vi "Set speed DSP402.vi"(8 "error in (no error)":errorcluster, 10 "RpM":i16, 11 "DSP402 in":refnum<class "DSP402.lvclass">) -> (0 "error out":errorcluster, 3 "DSP402 out":refnum<class "DSP402.lvclass">)   [LabVIEW 2026, in "canopen_.lvlib" / "DSP402.lvclass"]
uses:
  DSP402.lvclass
  DSP402.lvclass/DSP402.ctl
  CANopen/Multiplexor.ctl
  CANopen Master.lvlib
  Download DSP402 (U32).vi
  Download DSP402 (U16).vi
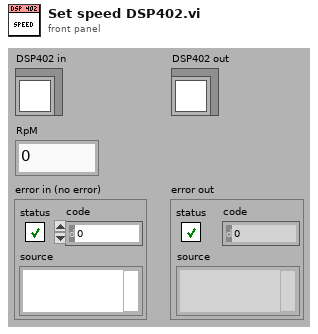
[diagram p1: front panel]
types:
  T1 = typedef "canopen.lvlib/DSP402.lvclass/DriveMode.ctl" = i8
  T2 = typedef "CANopen Master.lvlib/Multiplexor.ctl" = cluster{"Index":u16, "Sub-Index":i16}
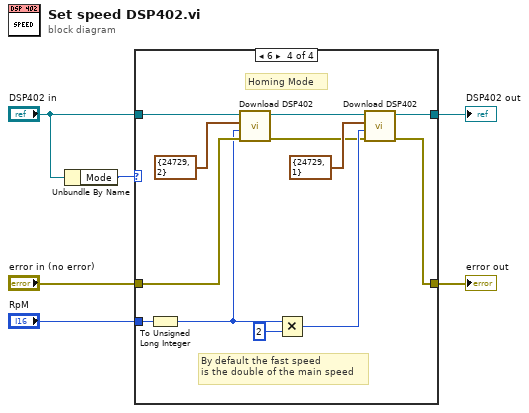
[diagram p0: block diagram]
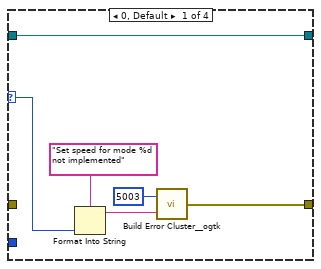
[diagram p2: hidden frame]
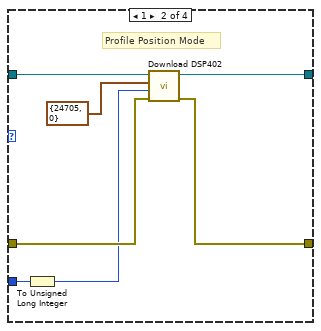
[diagram p3: hidden frame]
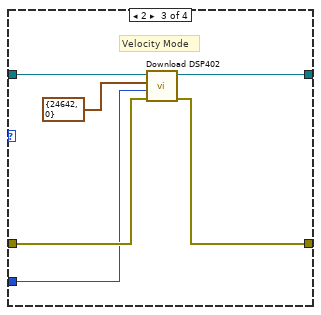
[diagram p4: hidden frame]
diagram:
  n1 = Unbundle By Name("DSP402 in") -> ("Mode"=w3:T1)
  n2 = case shown="6" w3 {
    selector: w3 -> [w9 _ _ _]
    tunnel: [w10 w18 w24 w30] -> w4
    tunnel: "error in (no error)" -> [_ w17 w23 w36]
    tunnel: "RpM" -> [_ w16 w22 w35]
    tunnel: [w7 w13 w20 w26] -> w2
    tunnel: "DSP402 in" -> [w7 w14 w21 w27]
    frame 0, Default {
      n3 = Format Into String(format string="Set speed for mode %d not implemented", w9) -> (resulting string=w11:string)  [unwired: 2 in, 1 out]
      n4 = call <userlib>:"Build Error Cluster__ogtk.vi"("String to Prepend to source (\"\")"=w11, "code"=5003) -> ("error out"=w10:errorcluster)
    }
    frame 1 {
      # "Profile Position Mode"
      n5 = To Unsigned Long Integer(number=w16) -> (unsigned 32bit integer=w15:u32)
      n6 = call-poly "Download DSP402.vi"("error in (no error)"=w17, "Value"=w15, "Multiplexor"=T2 {"Index"=24705, "Sub-Index"=0}, "DSP402 in"=w14) -> ("error out"=w18:errorcluster, "DSP402 out"=w13:refnum<class "DSP402.lvclass">)  [unwired: 1 in, 1 out]
    }
    frame 2 {
      # "Velocity Mode"
      n7 = call-poly "Download DSP402.vi"("error in (no error)"=w23, "Value"=w22, "Multiplexor"=T2 {"Index"=24642, "Sub-Index"=0}, "DSP402 in"=w21) -> ("error out"=w24:errorcluster, "DSP402 out"=w20:refnum<class "DSP402.lvclass">)  [unwired: 1 in, 1 out]
    }
    frame 6 {
      # "By default the fast speed\nis the double of the main speed"
      # "Homing Mode"
      n8 = To Unsigned Long Integer(number=w35) -> (unsigned 32bit integer=w34:u32)
      n9 = call-poly "Download DSP402.vi"("error in (no error)"=w36, "Value"=w34, "Multiplexor"=T2 {"Index"=24729, "Sub-Index"=2}, "DSP402 in"=w27) -> ("error out"=w29:errorcluster, "DSP402 out"=w28:refnum<class "DSP402.lvclass">)  [unwired: 1 in, 1 out]
      n10 = Multiply(x=w34, y=u32 2) -> (x*y=w32:u32)
      n11 = call-poly "Download DSP402.vi"("error in (no error)"=w29, "Value"=w32, "Multiplexor"=T2 {"Index"=24729, "Sub-Index"=1}, "DSP402 in"=w28) -> ("error out"=w30:errorcluster, "DSP402 out"=w26:refnum<class "DSP402.lvclass">)  [unwired: 1 in, 1 out]
    }
  }
  "error out" <- w4
  "DSP402 out" <- w2
